vi "UnlockBuffers.vi"(8 "error in":errorcluster, 9 "ms timeout (-1)":i32=-1, 10 "ptrs in":u64[](array[numeric])) -> (0 "error out":errorcluster)   [LabVIEW 2016]
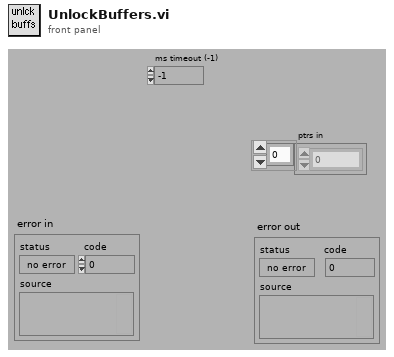
[diagram p1: front panel]
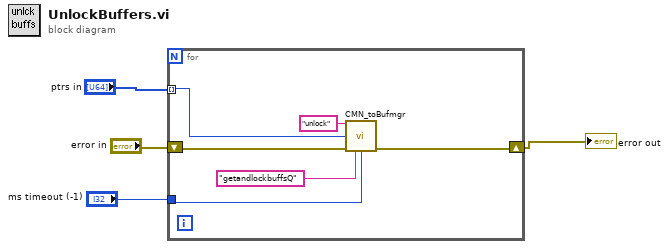
[diagram p0: block diagram]
diagram:
  n1 = for {
    shift-right: [w9] -> w2
    shift-left: "error in" -> [w10]
    tunnel: "ms timeout (-1)" -> [w8]
    tunnel: "ptrs in" -> [w5] mode=indexing
    n2 = call "CMN_toBufmgr.vi"("command"="unlock", "bufpointer"=w5, "error in"=w10, "responseQ"="getandlockbuffsQ", "ms timeout (-1)"=w8) -> ("error out"=w9:errorcluster)  [unwired: 3 in, 7 out]
  }
  "error out" <- w2
